vi "demo.vi"() -> ()   [LabVIEW 2012]
uses:
  FIFO(STR).lvclass
panel:
  in  "停止":bool
  out "采集数据表":string[][](table)
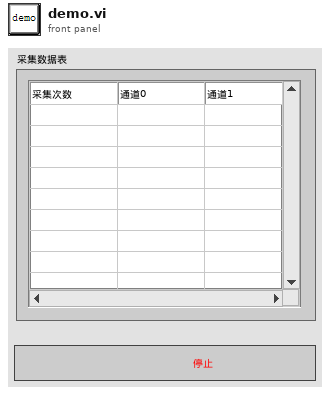
[diagram p1: front panel]
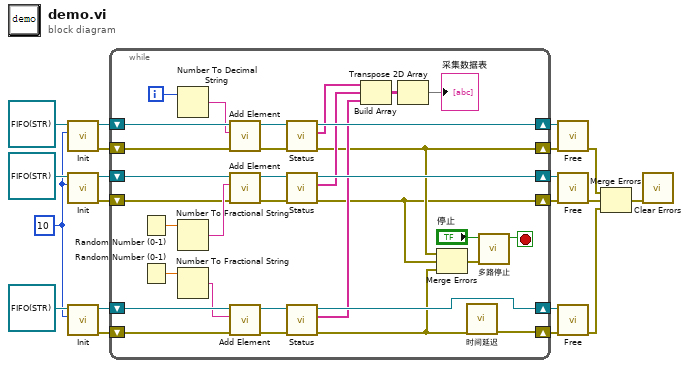
[diagram p0: block diagram]
diagram:
  w12 = 10 ("size")
  n1 = call "Init.vi"("size"=w12, "FIFO in"=refnum<class "FIFO(STR).lvclass"> refnum ("FIFO(STR).lvclass")) -> ("error out"=w11:errorcluster, "FIFO out"=w18:refnum<class "FIFO(STR).lvclass">)  [unwired: 8 in]
  n2 = call "Init.vi"("size"=w12, "FIFO in"=refnum<class "FIFO(STR).lvclass"> refnum) -> ("error out"=w10:errorcluster, "FIFO out"=w17:refnum<class "FIFO(STR).lvclass">)  [unwired: 8 in]
  n3 = call "Init.vi"("size"=w12, "FIFO in"=refnum<class "FIFO(STR).lvclass"> refnum) -> ("error out"=w9:errorcluster, "FIFO out"=w1:refnum<class "FIFO(STR).lvclass">)  [unwired: 8 in]
  n4 = while {
    shift-right: [w46] -> w16
    shift-left: w18 -> [w53]
    shift-right: [w44] -> w15
    shift-left: w17 -> [w49]
    shift-right: [w37] -> w13
    shift-left: w1 -> [w39]
    shift-right: [w26] -> w3
    shift-left: w11 -> [w33]
    shift-right: [w25] -> w2
    shift-left: w10 -> [w31]
    shift-right: [w22] -> w8
    shift-left: w9 -> [w29]
    i -> [w52]
    stop <- w23 stop-if-true
    n5 = Random Number (0-1)() -> (number: 0 to 1=w50:dbl)
    n6 = Random Number (0-1)() -> (number: 0 to 1=w35:dbl)
    n7 = Number To Decimal String(number=w52) -> (decimal integer string=w51:string)  [unwired: 1 in]
    n8 = Number To Fractional String(number=w50) -> (F-format string=w48:string)  [unwired: 3 in]
    n9 = Number To Fractional String(number=w35) -> (F-format string=w34:string)  [unwired: 3 in]
    n10 = call "Add Element.vi"("error in (no error)"=w33, "Element"=w51, "FIFO in"=w53) -> ("error out"=w32:errorcluster, "FIFO out"=w47:refnum<class "FIFO(STR).lvclass">)  [unwired: 6 in, 1 out]
    n11 = call "Add Element.vi"("error in (no error)"=w31, "Element"=w48, "FIFO in"=w49) -> ("error out"=w30:errorcluster, "FIFO out"=w45:refnum<class "FIFO(STR).lvclass">)  [unwired: 6 in, 1 out]
    n12 = call "Add Element.vi"("error in (no error)"=w29, "Element"=w34, "FIFO in"=w39) -> ("error out"=w28:errorcluster, "FIFO out"=w38:refnum<class "FIFO(STR).lvclass">)  [unwired: 6 in, 1 out]
    n13 = call "Status.vi"("error in (no error)"=w32, "FIFO in"=w47) -> ("error out"=w26:errorcluster, "Current Elements"=w41:string[], "FIFO out"=w46:refnum<class "FIFO(STR).lvclass">)  [unwired: 6 in, 1 out]
    n14 = call "Status.vi"("error in (no error)"=w30, "FIFO in"=w45) -> ("error out"=w25:errorcluster, "Current Elements"=w40:string[], "FIFO out"=w44:refnum<class "FIFO(STR).lvclass">)  [unwired: 6 in, 1 out]
    n15 = call "Status.vi"("error in (no error)"=w28, "FIFO in"=w38) -> ("error out"=w21:errorcluster, "Current Elements"=w36:string[], "FIFO out"=w37:refnum<class "FIFO(STR).lvclass">)  [unwired: 6 in, 1 out]
    n16 = Build Array(w41, w40, w36) -> (w43:string[][])
    n17 = Transpose 2D Array(2D array=w43) -> (transposed array=→"采集数据表":string[][])
    n18 = Merge Errors(w26, w25, w21) -> (w24:errorcluster)
    n19 = call "时间延迟"("error in (no error)"=w21) -> ("error out"=w22:errorcluster)  [unwired: 10 in]
    n20 = call "多路停止.vi"("error in (no error)"=w24, "停止"="停止") -> ("为真停止"=w23:bool)  [unwired: 6 in, 2 out]
  }
  n21 = call "Free.vi"("error in (no error)"=w3, "FIFO in"=w16) -> ("error out"=w7:errorcluster)  [unwired: 9 in]
  n22 = call "Free.vi"("error in (no error)"=w2, "FIFO in"=w15) -> ("error out"=w6:errorcluster)  [unwired: 9 in]
  n23 = call "Free.vi"("error in (no error)"=w8, "FIFO in"=w13) -> ("error out"=w5:errorcluster)  [unwired: 9 in]
  n24 = Merge Errors(w7, w6, w5) -> (w4:errorcluster)
  n25 = call <vilib>:"Clear Errors.vi"("error in (no error)"=w4) -> ()  [unwired: 6 in, 1 out]
